vi "goToAngle.vi"() -> (2 "x2":dbl=0.003082 format="%.2f")   [LabVIEW 2020]
uses:
  <vilib>/Rock Robotics/WPI/ThirdParty/Sensors/navX/_TypeDefs/FRIC_navX_DeviceNumbersTypeDef.ctl
  Robot Global Data.vi
  <vilib>/addons/control/pid/pid.llb/PID (DBL).vi
  <vilib>/addons/control/pid/NI_PID_pid.lvlib
panel:
  in  "invert":dbl=1.0
  in  "PID gains":T1={"proportional gain (Kc)"=0.0067, "integral time (Ti, min)"=0.0, "derivative time (Td, min)"=0.0} {"derivative time (Td, min)" format="%.3f"; "integral time (Ti, min)" format="%.20f"; "proportional gain (Kc)" format="%.20f"}
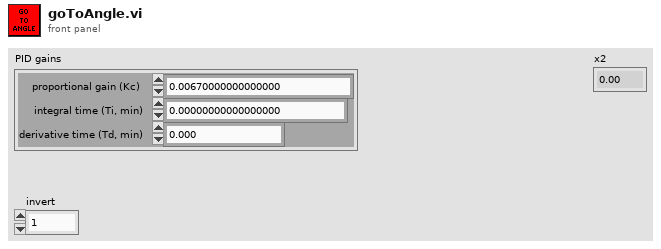
[diagram p1: front panel]
types:
  T1 = cluster{"proportional gain (Kc)":dbl, "integral time (Ti, min)":dbl, "derivative time (Td, min)":dbl}
  T2 = typedef "FRIC_navX_DeviceNumbersTypeDef.ctl" = enum16{"Dev0", "Dev1", "Dev2", "Dev3"}
  T3 = cluster{"Rollover":dbl, "Yaw":dbl, "Cont Yaw":dbl}
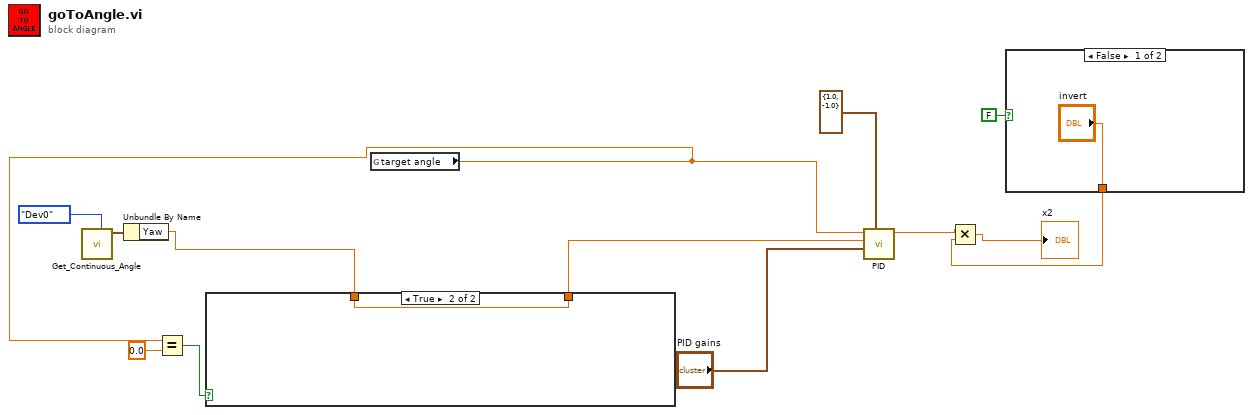
[diagram p0: block diagram]
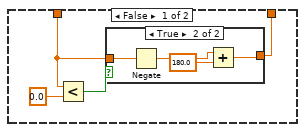
[diagram p2: hidden frame]
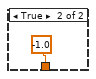
[diagram p4: hidden frame]
diagram:
  n1 = call <vilib>:"Get_Continuous_Angle.vi"("Device Number"=FRIC_navX_DeviceNumbersTypeDef."Dev0") -> ("Continuous Angle"=w8:T3)  [unwired: 10 in]
  n2 = Unbundle By Name(w8) -> ("Yaw"=w1:dbl)
  n3 = global read "Robot Global Data.vi" "target angle"() -> (w4:dbl)
  n4 = Equal?(x=w4, y=0.0) -> (x = y?=w5:bool)
  n5 = case shown="True" w5 {
    tunnel: w1 -> [w15 w23]
    tunnel: [w14 w23] -> w2
    frame False {
      n6 = Less?(x=w15, y=0.0) -> (x < y?=w17:bool)
      n7 = case shown="True" w17 {
        tunnel: w15 -> [w18 w22]
        tunnel: [w18 w19] -> w14
        frame False {
        }
        frame True {
          n8 = Negate(x=w22) -> (-x=w21:dbl)
          n9 = Add(x=w21, y=180.0) -> (x+y=w19:dbl)
        }
      }
    }
    frame True {
    }
  }
  n10 = call-poly <vilib>:"PID.vi"("output range"=cluster{"output high":dbl, "output low":dbl} {"output high"=1.0, "output low"=-1.0}, "PID gains"="PID gains", "process variable"=w2, "setpoint"=w4) -> ("output"=w10:dbl)  [unwired: 6 in, 1 out]
  n11 = case shown="False" FALSE {
    tunnel: ["invert" -1.0 ("invert")] -> w9
    frame False {
    }
    frame True {
    }
  }
  n12 = Multiply(x=w10, y=w9) -> (x*y=→"x2":dbl)
